vi "OAT Order Magnitude and Phase Plot(XY) (Multi Channels).vi"(6 "X axis selection":u16(ring)=2 items=["Time", "Revolution", "RPM"], 7 "reset? (True)":bool=TRUE, 8 "speed profile":T1 {"speed [RPM]" format="%.2f"; "time [s]" format="%.2f"}, 9 "samples/rev":dbl=1.0 format="%.2f", 10 "phase lag  (even angular)":dbl[][][](array[numeric]) format="%.2f", 11 "magnitudes (even angular)":dbl[][][](array[numeric]) format="%.2f") -> (1 "X unit":string, 2 "phase lag":cluster{"X":dbl[], "Y":dbl[]}[][](array[cluster]) {"Y" format="%.2f"; "X" format="%.2f"}, 3 "magnitudes":cluster{"X":dbl[], "Y":dbl[]}[][](array[cluster]) {"Y" format="%.2f"; "X" format="%.2f"})   [LabVIEW 2017, in "SoundVib_Resampling.lvlib"]
uses:
  <vilib>/addons/Sound and Vibration/Order Analysis/Resample Order Tracking/SoundVib_Resampling.lvlib
  <vilib>/addons/Sound and Vibration/Order Analysis/Tach Process/SubVIs/speed profile.ctl
  <vilib>/Analysis/1siggen.llb/Ramp Pattern by Samples.vi
  <vilib>/Analysis/NI_AALBase.lvlib
  <vilib>/addons/Sound and Vibration/Order Analysis/Tach Process/SoundVib_TachProcess.lvlib
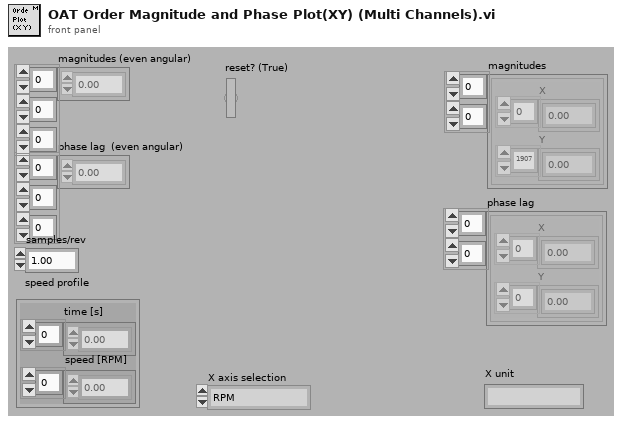
[diagram p1: front panel]
types:
  T1 = typedef "SoundVib_TachProcess.lvlib/speed profile.ctl" = cluster{"time [s]":dbl[], "speed [RPM]":dbl[]}
  T2 = cluster{"speed [RPM]":dbl[], "magnitudes (even angular)":dbl[]}
  T3 = cluster{"speed [RPM]":dbl[], "phase lag  (even angular)":dbl[]}
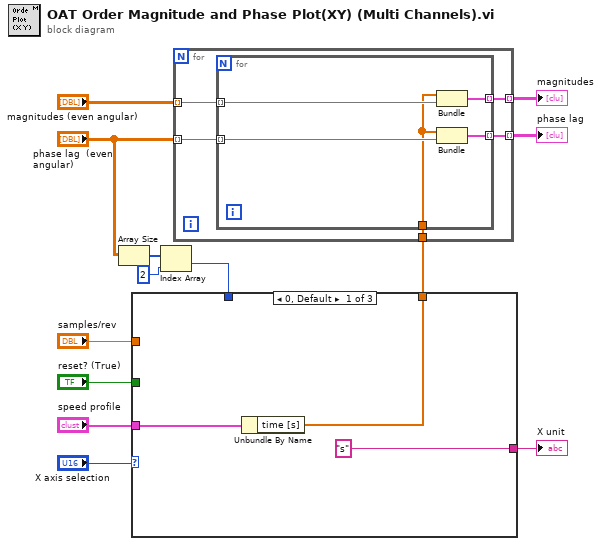
[diagram p0: block diagram]
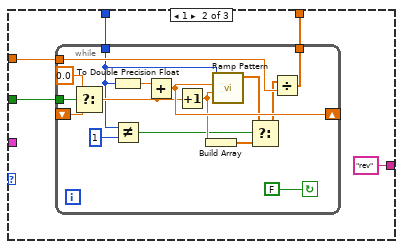
[diagram p2: hidden frame]
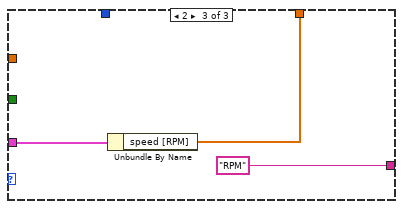
[diagram p3: hidden frame]
diagram:
  n1 = Array Size(array="phase lag  (even angular)") -> (size(s)=w9:i32[])
  n2 = Index Array(array=w9, index=2) -> (element=w6:i32)
  n3 = case shown="0, Default" "X axis selection" {
    tunnel: "speed profile" -> [w16 _ w40]
    tunnel: [w15 w20 w39] -> w7
    tunnel: w6 -> [_ w19 _]
    tunnel: "samples/rev" -> [_ w18 _]
    tunnel: ["s" "rev" "RPM"] -> w4
    tunnel: "reset? (True)" -> [_ w17 _]
    frame 0, Default {
      n4 = Unbundle By Name(w16) -> ("time [s]"=w15:dbl[])
    }
    frame 1 {
      n5 = while {
        tunnel: [w37] -> w20
        tunnel: w18 -> [w36]
        tunnel: w17 -> [w34]
        shift-right: [w31] -> _
        shift-left: _ -> [w32]
        tunnel: w19 -> [w28]
        stop <- FALSE continue-if-true
        n6 = Select(t=0.0 ("f"), s=w34, f=w32) -> (s? t:f=w30:dbl)
        n7 = To Double Precision Float(number=w28) -> (double precision float=w22:dbl)
        n8 = Not Equal?(x=w28, y=1) -> (x != y?=w26:bool)
        n9 = Add(x=w22, y=w30) -> (x+y=w31:dbl)
        n10 = Increment(x=w30) -> (x+1=w27:dbl)
        n11 = Build Array(w27) -> (w24:dbl[])
        n12 = call-poly <vilib>:"Ramp Pattern.vi"("start"=w27, "end"=w31, "samples"=w28) -> ("Ramp Pattern"=w25:dbl[])  [unwired: 7 in, 1 out]
        n13 = Select(t=w25, s=w26, f=w24) -> (s? t:f=w23:dbl[])
        n14 = Divide(x=w23, y=w36) -> (x/y=w37:dbl[])
      }
    }
    frame 2 {
      n15 = Unbundle By Name(w40) -> ("speed [RPM]"=w39:dbl[])
    }
  }
  "X unit" <- w4
  n16 = for {
    tunnel: "magnitudes (even angular)" -> [w45] mode=indexing
    tunnel: "phase lag  (even angular)" -> [w44] mode=indexing
    tunnel: w7 -> [w43]
    tunnel: [w42] -> w2 mode=indexing
    tunnel: [w41] -> w1 mode=indexing
    n17 = for {
      tunnel: w44 -> [w47] mode=indexing
      tunnel: [w49] -> w41 mode=indexing
      tunnel: [w50] -> w42 mode=indexing
      tunnel: w45 -> [w48] mode=indexing
      tunnel: w43 -> [w46]
      n18 = Bundle("speed [RPM]"=w46, "magnitudes (even angular)"=w48) -> (w50:T2)  [unwired: 1 in]
      n19 = Bundle("speed [RPM]"=w46, "phase lag  (even angular)"=w47) -> (w49:T3)  [unwired: 1 in]
    }
  }
  "phase lag" <- w1
  "magnitudes" <- w2
